vi "SmoothPath.vi"(4 "ball":T1, 6 "Initial State":dbl[](array[numeric]), 7 "Robot in":T2={"id"=0, "function"=enum."Attacker", "x"=0.0, "y"=0.0, "orientation"=0.0, "v_tangent"=0.0, "v_normal"=0.0, "v_ang"=0.0, "kick_x"=0.0, "kick_z"=0.0, "dribble"=FALSE, "Timestamp"=timestamp(0 s since 1904-01-01), "estimatives"={"est_v_tangent"=0.0, "est_v_normal"=0.0, "est_vx"=0.0, "est_vy"=0.0, "Pos Robot Est"=[]}, "dest_x_kick"=0.0, "dest_y_kick"=0.0, "Gap Coord"=[], "States"=enum."GoToTangent", "Path "=[], "Path  Smooth"=[], "Dest"=[]}, 8 "our_robots":T2[](array[typedef]), 9 "enemy_robots":T2[](array[typedef]), 10 "Path":dbl[][](array[numeric]), 11 "Goal":dbl[](array[numeric])) -> (2 "SmoothPath":dbl[][](array[numeric]))   [LabVIEW 2018]
uses:
  Core/AI Robot.ctl
  Intel/Functions Enum.ctl
  Intel/AttackerStates.ctl
  PathDests.ctl
  PathDest.ctl
  Core/AI Ball.ctl
panel:
  out "appended array":dbl[][](array[numeric])
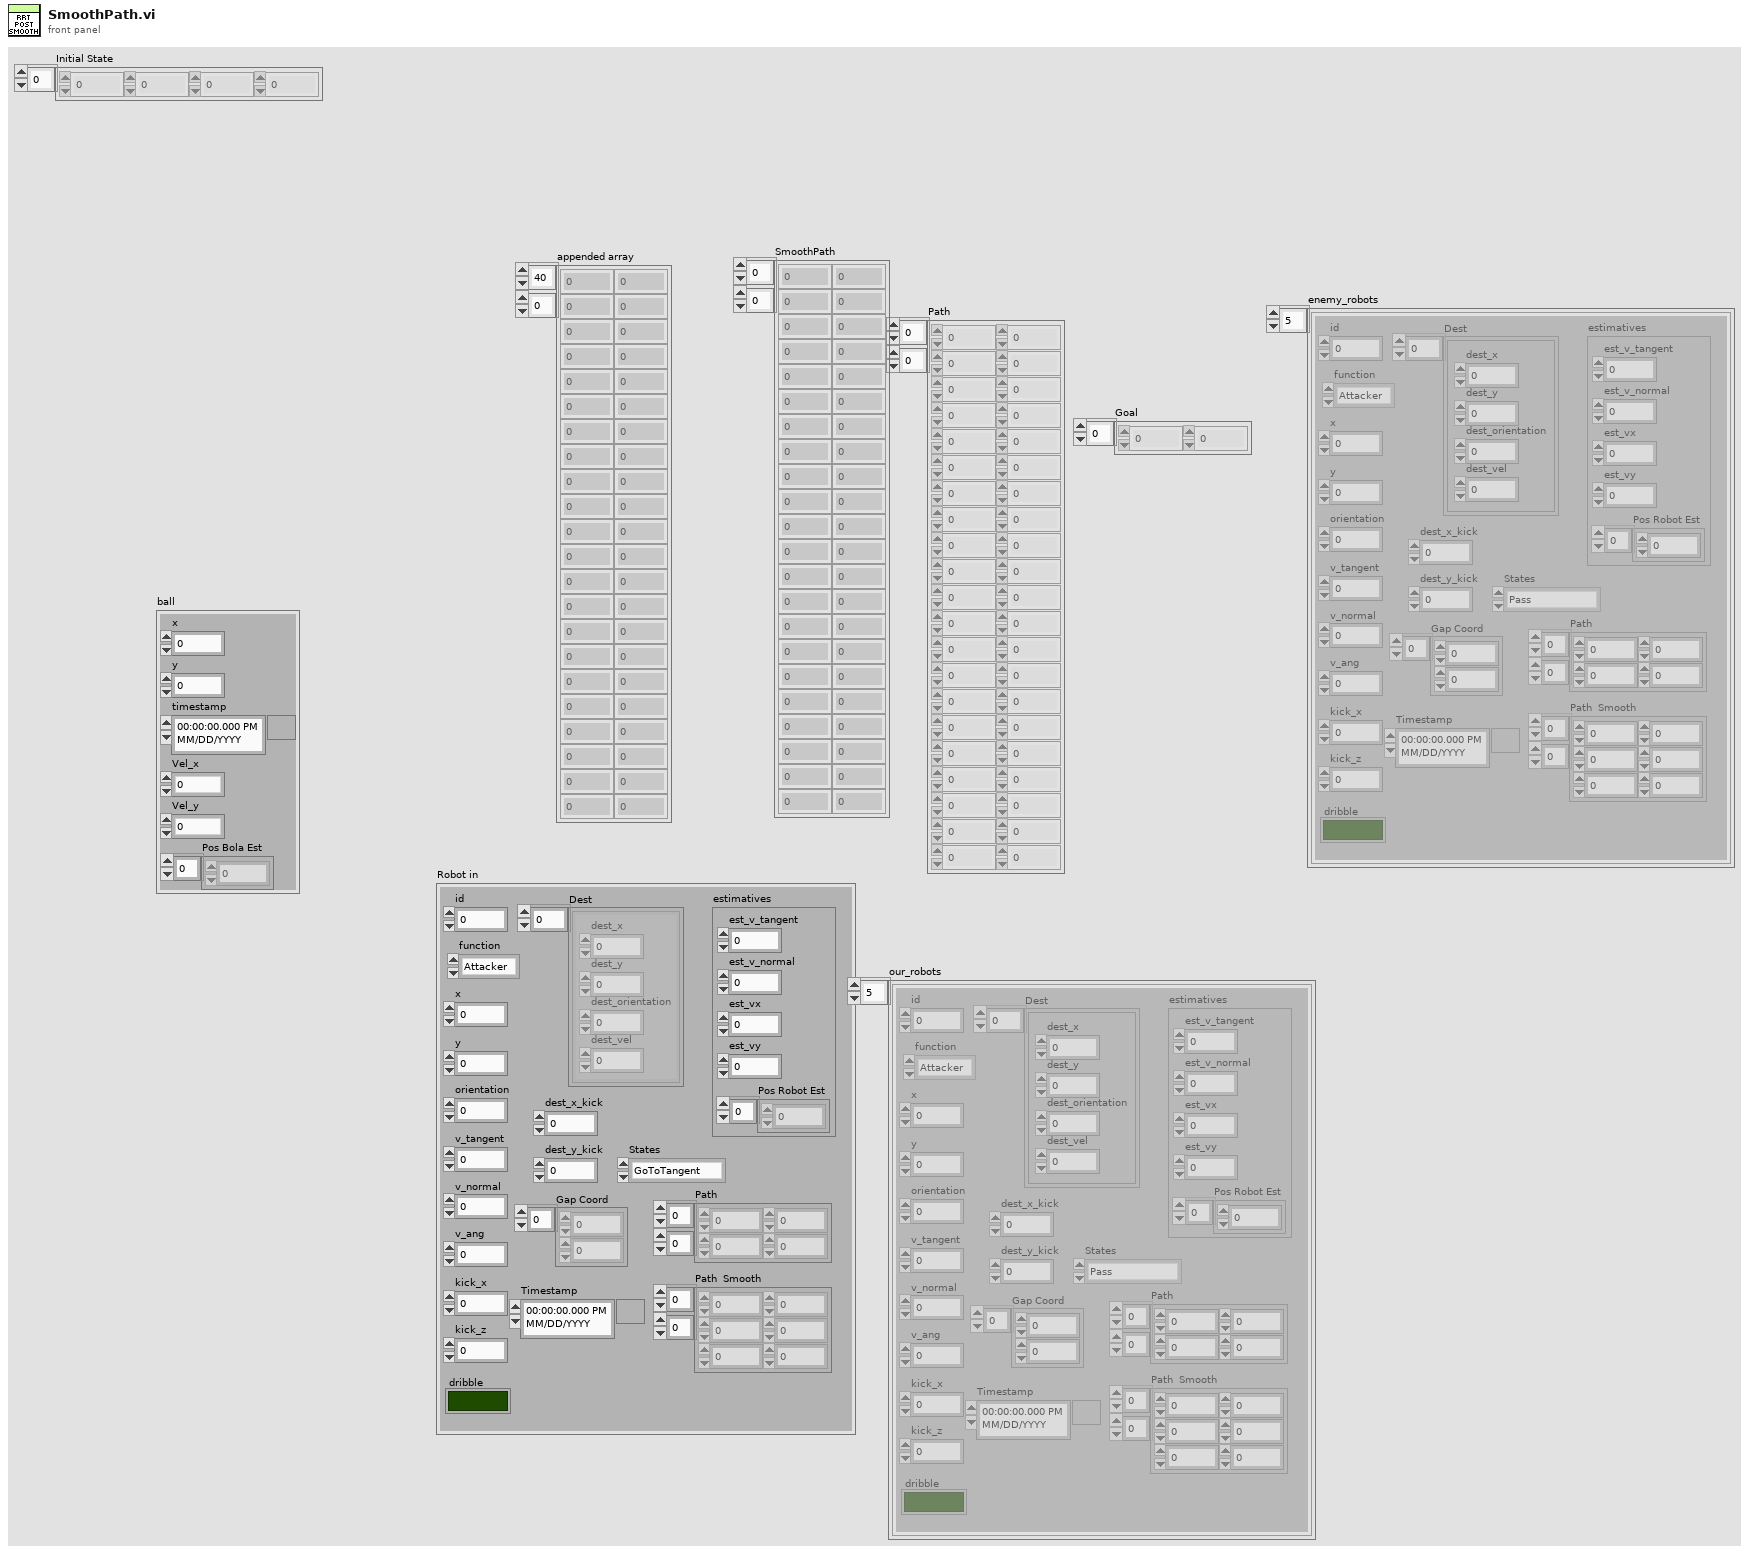
[diagram p1: front panel]
types:
  T1 = typedef "AI Ball.ctl" = cluster{"x":dbl, "y":dbl, "timestamp":timestamp, "Vel_x":dbl, "Vel_y":dbl, "Pos Bola Est":dbl[]}
  T2 = typedef "AI Robot.ctl" = cluster{"id":u32, "function":T3, "x":dbl, "y":dbl, "orientation":dbl, "v_tangent":dbl, "v_normal":dbl, "v_ang":dbl, "kick_x":dbl, "kick_z":dbl, "dribble":bool, "Timestamp":timestamp, "estimatives":cluster{"est_v_tangent":dbl, "est_v_normal":dbl, "est_vx":dbl, "est_vy":dbl, "Pos Robot Est":dbl[]}, "dest_x_kick":dbl, "dest_y_kick":dbl, "Gap Coord":dbl[], "States":T4, "Path ":dbl[][], "Path  Smooth":dbl[][], "Dest":T5}
  T3 = typedef "Functions Enum.ctl" = enum16{"Attacker", "Goalie", "Defender", "Striker", "Goto 0", "Dummy", "Kicker", "ZigZag"}
  T4 = typedef "AttackerStates.ctl" = enum16{"Pass", "GoToTangent", "BallGetting", "GoToKick", "Rotate anti-clockwise", "Rotate Clockwise", ""}
  T5 = typedef "PathDests.ctl" = T6[]
  T6 = typedef "PathDest.ctl" = cluster{"dest_x":dbl, "dest_y":dbl, "dest_orientation":dbl, "dest_vel":dbl}
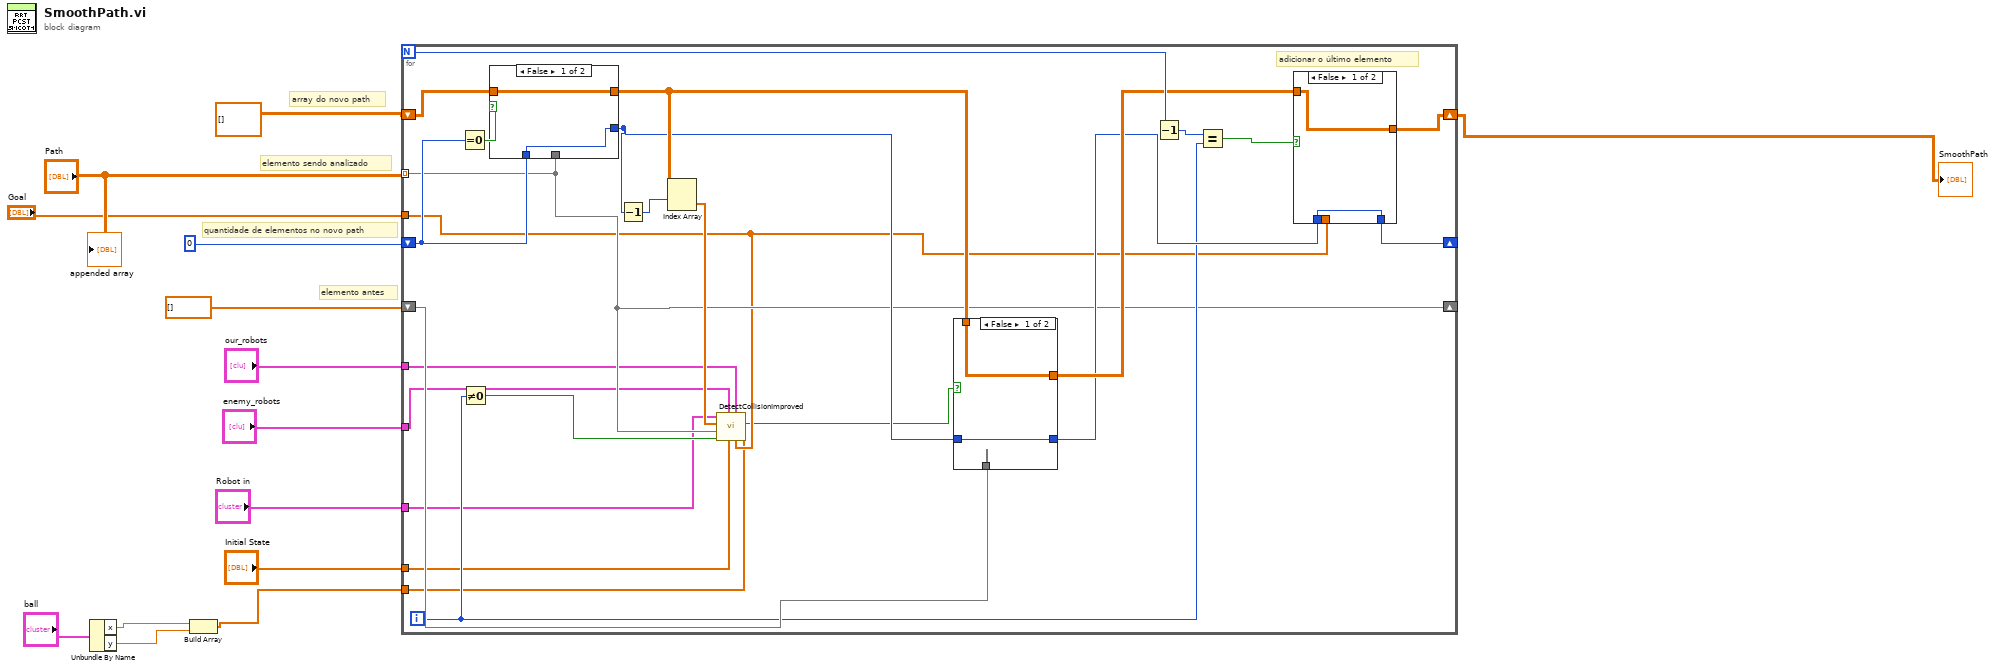
[diagram p0: block diagram]
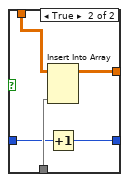
[diagram p2: hidden frame]
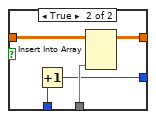
[diagram p3: hidden frame]
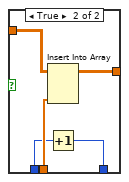
[diagram p4: hidden frame]
diagram:
  # "elemento sendo analizado"
  # "quantidade de elementos no novo path"
  # "elemento antes"
  # "array do novo path"
  n1 = Unbundle By Name("ball") -> ("x"=w2:dbl, "y"=w1:dbl)
  n2 = Build Array(w2, w1) -> (w4:dbl[])
  n3 = for {
    N -> [w37]
    tunnel: "Path" -> [w21] mode=indexing
    tunnel: "enemy_robots" -> [w19]
    shift-right: [w31] -> w5
    shift-left: dbl[][] [] ("Path") -> [w35]
    shift-right: [w21] -> _
    shift-left: dbl[] [] ("Path") -> [w25]
    shift-right: [w30] -> _
    shift-left: 0 -> [w34]
    tunnel: "Robot in" -> [w20]
    tunnel: "Goal" -> [w18]
    tunnel: "Initial State" -> [w22]
    tunnel: "our_robots" -> [w16]
    tunnel: w4 -> [w15]
    i -> [w23]
    # "adicionar o último elemento"
    n4 = Equal To 0?(x=w34) -> (x = 0?=w36:bool)
    n5 = Not Equal To 0?(x=w23) -> (x != 0?=w24:bool)
    n6 = case shown="False" w36 {
      tunnel: w21 -> [_ w53]
      tunnel: w35 -> [w47 w52]
      tunnel: [w47 w51] -> w29
      tunnel: w34 -> [w48 w50]
      tunnel: [w48 w49] -> w27
      frame False {
      }
      frame True {
        n7 = Increment(x=w50) -> (x+1=w49:i32)
        n8 = Insert Into Array(array=w52, new element=w53) -> (w51:dbl[][])  [unwired: 2 in]
      }
    }
    n9 = Decrement(x=w27) -> (x-1=w33:i32)
    n10 = Index Array(array=w29, index (row)=w33) -> (element=w32:dbl[])  [unwired: 1 in]
    n11 = call "DetectCollisionImproved.vi"("ball"=w15, "Goal"=w18, "our_robots"=w16, "Initial State"=w22, "enemy_robots"=w19, "Is not first robot?"=w24, "element being analyzed"=w21, "element already in path"=w32, "Robot in"=w20) -> ("Is there colision?"=w17:bool)  [unwired: 2 in]
    n12 = case shown="False" w17 {
      tunnel: w25 -> [_ w46]
      tunnel: [w40 w45] -> w28
      tunnel: w29 -> [w40 w44]
      tunnel: w27 -> [w41 w43]
      tunnel: [w41 w42] -> w26
      frame False {
      }
      frame True {
        n13 = Insert Into Array(array=w44, new element=w46) -> (w45:dbl[][])  [unwired: 2 in]
        n14 = Increment(x=w43) -> (x+1=w42:i32)
      }
    }
    n15 = Decrement(x=w37) -> (x-1=w38:i32)
    n16 = Equal?(x=w38, y=w23) -> (x = y?=w39:bool)
    n17 = case shown="False" w39 {
      tunnel: w18 -> [_ w60]
      tunnel: w28 -> [w55 w59]
      tunnel: [w55 w58] -> w31
      tunnel: w26 -> [w54 w57]
      tunnel: [w54 w56] -> w30
      frame False {
      }
      frame True {
        n18 = Insert Into Array(array=w59, new element=w60) -> (w58:dbl[][])  [unwired: 2 in]
        n19 = Increment(x=w57) -> (x+1=w56:i32)
      }
    }
  }
  "SmoothPath" <- w5
  "appended array" <- "Path"
